vi "Get Digital Gain (Pre).vi"(2 "gen":refnum<class "niUSRP Tx DSP v2 FPGA.lvclass">, 11 "ch":u8) -> (4 "digital gain":refnum<class "Digital Gain Interface (IQ 18-bit).lvclass">)   [LabVIEW 2025, in "niUSRP Tx DSP v2 FPGA.lvclass"]
uses:
  niUSRP Tx DSP v2 FPGA.lvclass
  <instrlib>/_niInstr/DSP Control/Interface/v1/FPGA/Digital Gain/IQ 18-bit/Digital Gain Interface (IQ 18-bit).lvclass
  niUSRP Tx DSP v2 FPGA.lvclass/niUSRP Tx DSP v2 FPGA.ctl
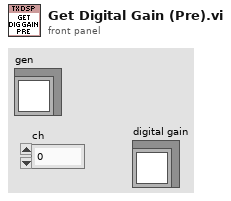
[diagram p1: front panel]
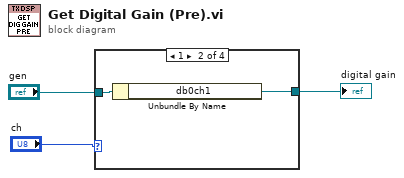
[diagram p0: block diagram]
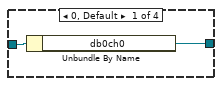
[diagram p2: hidden frame]
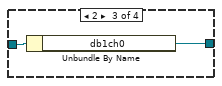
[diagram p3: hidden frame]
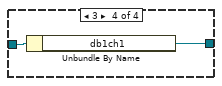
[diagram p4: hidden frame]
diagram:
  n1 = case shown="1" "ch" {
    tunnel: "gen" -> [w5 w7 w9 w11]
    tunnel: [w4 w6 w8 w10] -> w2
    frame 0, Default {
      n2 = Unbundle By Name(w5) -> ("db0ch0"=w4:refnum<class "Digital Gain Interface (IQ 18-bit).lvclass">)
    }
    frame 1 {
      n3 = Unbundle By Name(w7) -> ("db0ch1"=w6:refnum<class "Digital Gain Interface (IQ 18-bit).lvclass">)
    }
    frame 2 {
      n4 = Unbundle By Name(w9) -> ("db1ch0"=w8:refnum<class "Digital Gain Interface (IQ 18-bit).lvclass">)
    }
    frame 3 {
      n5 = Unbundle By Name(w11) -> ("db1ch1"=w10:refnum<class "Digital Gain Interface (IQ 18-bit).lvclass">)
    }
  }
  "digital gain" <- w2
